vi "NMLAddress2VISA.vi"(1 "NML Address":string) -> (0 "VISA resource name":refnum<visa-resource-name>)   [LabVIEW 2021]
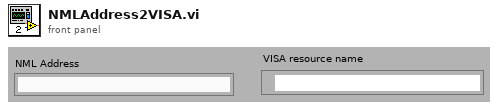
[diagram p1: front panel]
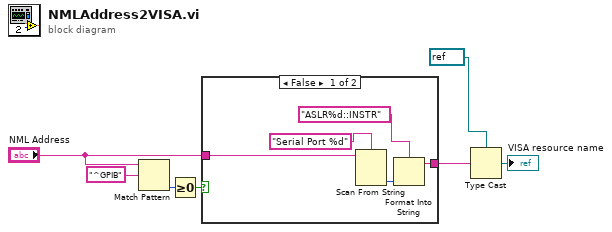
[diagram p0: block diagram]
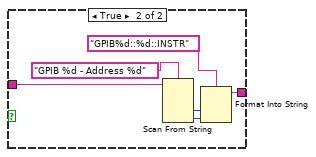
[diagram p2: hidden frame]
diagram:
  n1 = Match Pattern(string="NML Address", regular expression="^GPIB") -> (offset past match=w5:i32)  [unwired: 1 in, 3 out]
  n2 = Greater Or Equal To 0?(x=w5) -> (x >= 0?=w6:bool)
  n3 = case shown="False" w6 {
    tunnel: [w12 w18] -> w3
    tunnel: "NML Address" -> [w9 w15]
    frame False {
      n4 = Scan From String(format string="Serial Port %d", input string=w9) -> (output 1=w8:i32)  [unwired: 3 in, 3 out]
      n5 = Format Into String(format string="ASLR%d::INSTR", w8) -> (resulting string=w12:string)  [unwired: 2 in, 1 out]
    }
    frame True {
      n6 = Scan From String(format string="GPIB %d - Address %d", input string=w15) -> (output 1=w14:i32, output 2=w13:i32)  [unwired: 4 in, 3 out]
      n7 = Format Into String(format string="GPIB%d::%d::INSTR", w14, w13) -> (resulting string=w18:string)  [unwired: 2 in, 1 out]
    }
  }
  n8 = Type Cast(type=refnum<visa-resource-name> refnum ("VISA resource name"), x=w3) -> (*(type *) &x=→"VISA resource name":refnum<visa-resource-name>)
